vi "getMainBoard.vi"(10 "Machine":string="QAMT20") -> (0 "Cnt":i32, 2 "array":string[][](array[string]))   [LabVIEW 2012]
uses:
  <vilib>/addons/database/Connection.llb/DB Tools Open Connec (Path).vi
  <vilib>/addons/database/Connection.llb/Conn Execute.vi
  <vilib>/addons/database/Recordset.llb/Rec Fetch Recordset Data (R).vi
  <vilib>/addons/database/Recordset.llb/Rec Destroy - Connection.vi
  <vilib>/addons/database/_DB Variant To Data/Database Variant To Data.xnode
  <vilib>/addons/database/NI_Database_API.lvlib
panel:
  out "concatenated string":string
  out "error out":errorcluster
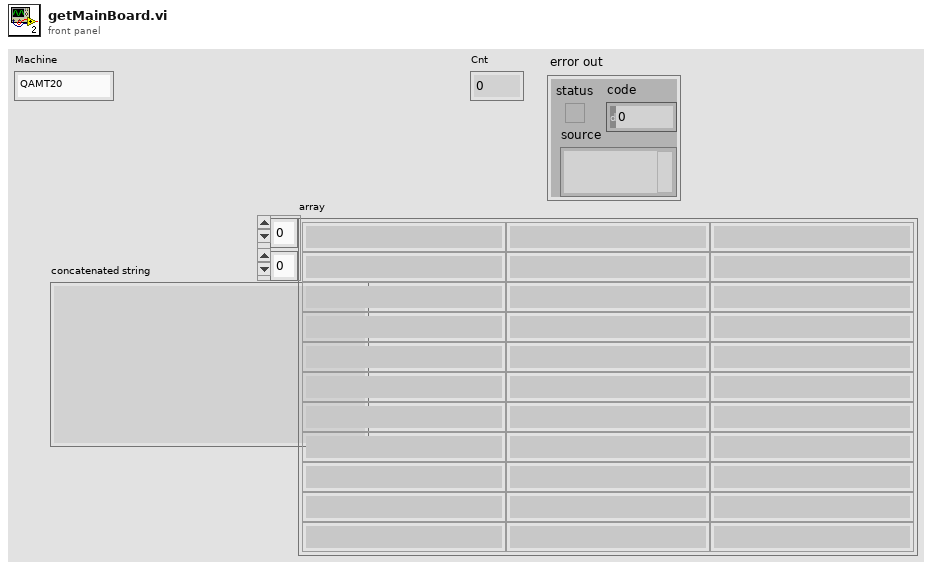
[diagram p1: front panel]
types:
  T1 = typedef "NI_Database_API.lvlib/Conn ObjectReference.ctl" = refnum<k1>
  T2 = typedef "NI_Database_API.lvlib/Rec ObjectReference.ctl" = refnum<k1>
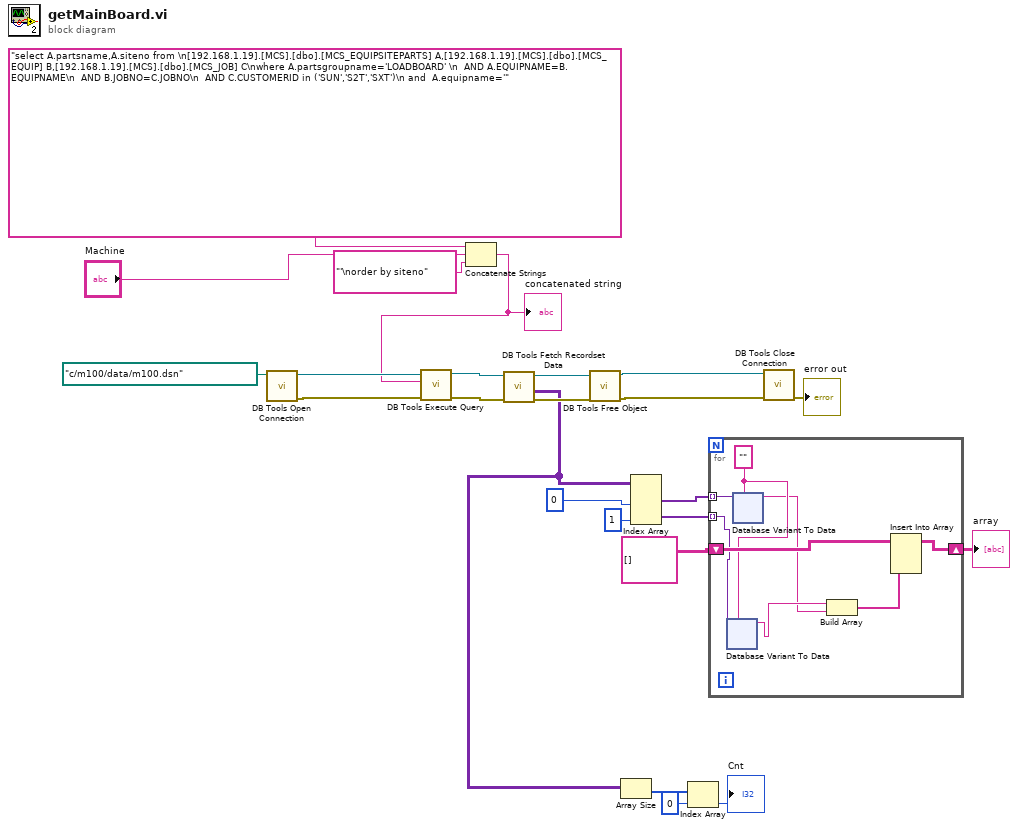
[diagram p0: block diagram]
diagram:
  n1 = call-poly <vilib>:"DB Tools Open Connection.vi"("connection information"=path "c:/m100/data/m100.dsn") -> ("error out"=w18:errorcluster, "connection reference"=w19:T1)  [unwired: 7 in]
  n2 = Concatenate Strings("select A.partsname,A.siteno from \n[192.168.1.19].[MCS].[dbo].[MCS_EQUIPSITEPARTS] A,[192.168.1.19].[MCS].[dbo].[MCS_EQUIP] B,[192.168.1.19].[MCS].[dbo].[MCS_JOB] C\nwhere A.partsgroupname='LOADBOARD' \n  AND A.EQUIPNAME=B.EQUIPNAME\n  AND B.JOBNO=C.JOBNO\n  AND C.CUSTOMERID in ('SUN','S2T','SXT')\n and  A.equipname='" ("SQL query"), "Machine", "'\norder by siteno" ("string")) -> (w11:string)
  "concatenated string" <- w11
  n3 = call-poly <vilib>:"DB Tools Execute Query.vi"("error in (no error)"=w18, "SQL query"=w11, "connection reference"=w19) -> ("error out"=w24:errorcluster, "recordset reference"=w23:T2)  [unwired: 5 in]
  n4 = call-poly <vilib>:"DB Tools Fetch Recordset Data.vi"("error in (no error)"=w24, "recordset reference"=w23) -> ("error out"=w21:errorcluster, "recordset data"=w4:variant[][], "recordset reference out"=w22:T2)  [unwired: 3 in]
  n5 = call-poly <vilib>:"DB Tools Free Object.vi"("error in (no error)"=w21, "recordset reference"=w22) -> ("error out"=w16:errorcluster, "connection reference"=w17:T1)  [unwired: 8 in]
  n6 = Array Size(array=w4) -> (size(s)=w3:i32[])
  n7 = Index Array(array=w4, index (col) #1=0 ("disabled index (col)"), index (col) #2=1 ("index (col)")) -> (element #1=w9:variant[], element #2=w6:variant[])  [unwired: 2 in]
  n8 = Index Array(array=w3, index=0) -> (element=→"Cnt":i32)
  n9 = for {
    tunnel: w9 -> [w32] mode=indexing
    shift-right: [w31] -> w5
    shift-left: string[][] [] ("array") -> [w30]
    tunnel: w6 -> [w29] mode=indexing
    w27 = ""
    n10 = xnode "Database Variant To Data"("database variant"=w29, "type"=w27) -> ("data"=w28:string)  [unwired: 1 in, 1 out]
    n11 = xnode "Database Variant To Data"("database variant"=w32, "type"=w27) -> ("data"=w26:string)  [unwired: 1 in, 1 out]
    n12 = Build Array(w28, w26) -> (w25:string[])
    n13 = Insert Into Array(array=w30, new element=w25) -> (w31:string[][])  [unwired: 2 in]
  }
  "array" <- w5
  n14 = call <vilib>:"DB Tools Close Connection.vi"("error in (no error)"=w16, "connection reference"=w17) -> ("error out"=→"error out":errorcluster)  [unwired: 5 in]
